vi "SVT FFT Spectrum (Complex).vi"   [LabVIEW 2017]
doc: "Computes the FFT spectrum of <B>scaled signal [EU]</B>. The VI returns FFT results as a <B>complex spectrum</B>. You can use this polymorphic VI to analyze data from a single channel or from N channels. The data type you wire to the <B>scaled signal [EU]</B> input determines the polymorphic instance to use."
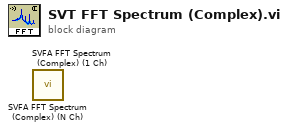
[diagram p0: block diagram]
diagram:
  n1 = call <vilib>:"SVFA FFT Spectrum (Complex) (N Ch).vi"() -> ()  [unwired: 16 in, 4 out]
  n2 = call <vilib>:"SVFA FFT Spectrum (Complex) (1 Ch).vi"() -> ()  [unwired: 16 in, 4 out]
